vi "DMR_Close.vi"() -> (0 "error code OUT":i32)   [LabVIEW 2014]
doc: "Frees internal data structures and decreases the usage counter for the device manager.\n\nThis VI frees internal memory previously allocated by the DMR_Init VI and decrements the internal usage counter. For each call to DMR_Init the user must call this VI once before ending the application again as otherwise resource leaks and other problems may arise.\n\nWhen the internal reference counter indicates, that the device manager is not needed anymore the device manager automatically closes all devices which still might be open.\n\nSee also:\nDMR_Init\n \nThe errorcode output will return 0 if successful or a negative error code of type otherwise. A list of valid error codes and their meaning can be found in the manual about this interface."
uses:
  mvDeviceManager.dll
panel:
  # "OUTPUT"
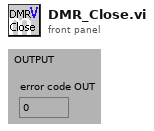
[diagram p1: front panel]
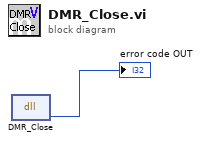
[diagram p0: block diagram]
diagram:
  n1 = dll-call lib="mvDeviceManager.dll" fn="DMR_Close"() -> (→"error code OUT":i32)  [unwired: 3 in, 2 out]
